vi "TranslateError.vi"(11 "error constant":errorcluster) -> (3 "error constant 2":errorcluster)   [LabVIEW 2026]
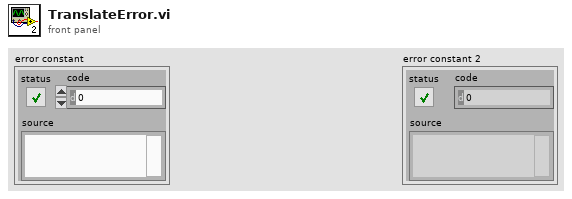
[diagram p1: front panel]
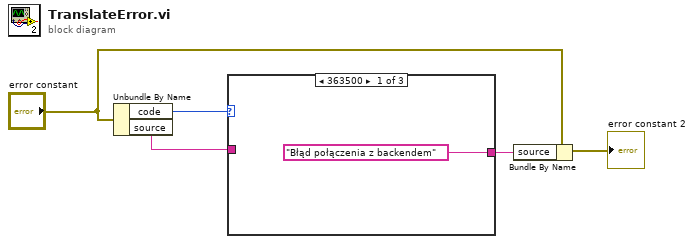
[diagram p0: block diagram]
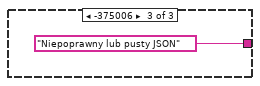
[diagram p3: hidden frame]
diagram:
  n1 = Unbundle By Name("error constant") -> ("code"=w5:i32, "source"=w1:string)
  n2 = case shown="363500" w5 {
    tunnel: ["Błąd połączenia z backendem" w7 "Niepoprawny lub pusty JSON"] -> w4
    tunnel: w1 -> [_ w7 _]
    frame 363500 {
    }
    frame 0, Default {
    }
    frame -375006 {
    }
  }
  n3 = Bundle By Name(cluster="error constant", "source"=w4) -> (→"error constant 2":errorcluster)
